vi "Filter-Get Spectrum.vi"(0 "Filter":T1 {"IIR Filter Cluster"."Forward Coefficients" format="%.4f"; "IIR Filter Cluster"."Reverse Coefficients" format="%.4f"}, 5 "Sampling Rate (Hz)":dbl, 7 "Npts":i32, 11 "error in (no error)":errorcluster) -> (4 "Filter out":T1 {"IIR Filter Cluster"."Forward Coefficients" format="%.4f"; "IIR Filter Cluster"."Reverse Coefficients" format="%.4f"}, 8 "spectrum":cdb[](array[numeric]), 15 "error out":errorcluster)   [LabVIEW 2020]
uses:
  Controls/Filter XCtl/Filter Data.ctl
  <vilib>/Analysis/2dsp.llb/Real FFT.vi
  <vilib>/Analysis/1siggen.llb/Ramp Pattern by Samples.vi
  <vilib>/Analysis/baseanly.llb/IIR Cascade Filter (DBL).vi
  Utility VIs/Math VIs/Linear to dB (array).vi
  <vilib>/Analysis/NI_AALBase.lvlib
  <vilib>/Analysis/NI_AALPro.lvlib
  Controls/Filter XCtl/Filter XCtl.xctl
panel:
  out "Magnitude":dbl[](graph)
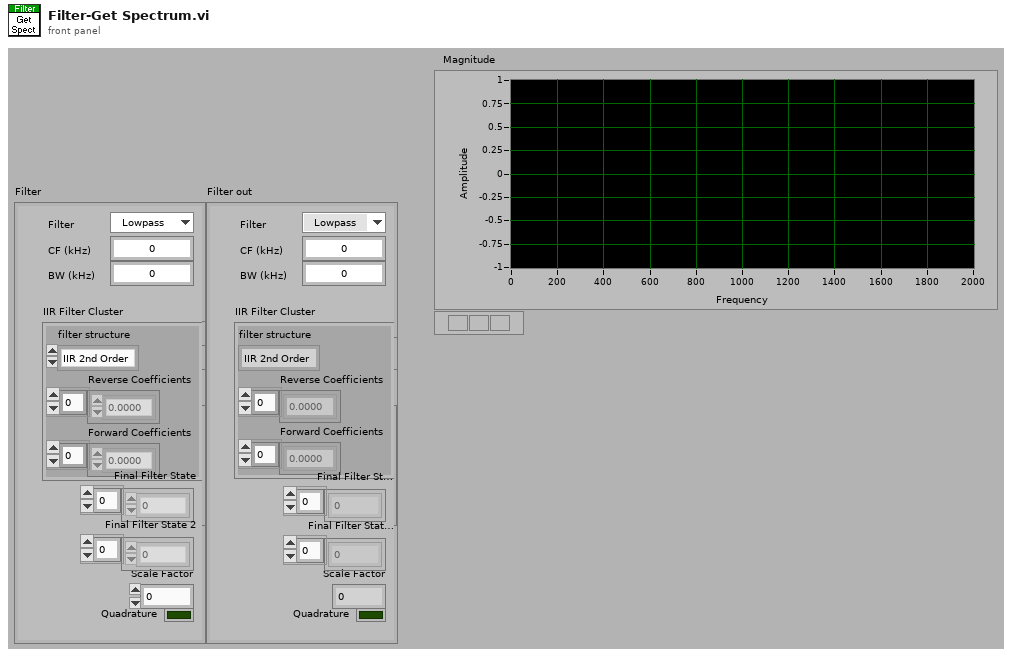
[diagram p1: front panel]
types:
  T1 = typedef "Filter XCtl.xctl/Filter Data.ctl" = cluster{"CF (kHz)":dbl, "BW (kHz)":dbl, "IIR Filter Cluster":cluster{"filter structure":enum32{"IIR 2nd Order", "IIR 4th Order"}, "Reverse Coefficients":dbl[], "Forward Coefficients":dbl[]}, "Final Filter State":dbl[], "Scale Factor":dbl, "Final Filter State 2":dbl[], "Quadrature":bool, "Type":enum16{"Lowpass", "Highpass", "Bandpass", "Bandstop", "OFF"}}
  T2 = enum16{"Lowpass", "Highpass", "Bandpass", "Bandstop", "OFF"}
  T3 = cluster{"filter structure":enum32{"IIR 2nd Order", "IIR 4th Order"}, "Reverse Coefficients":dbl[], "Forward Coefficients":dbl[]}
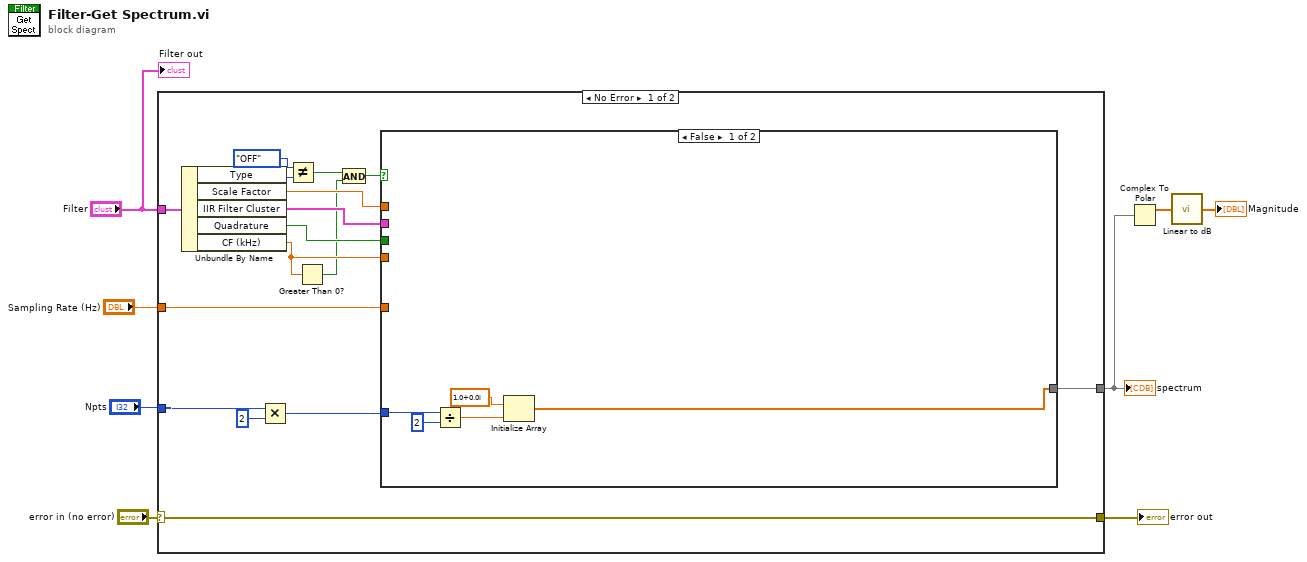
[diagram p0: block diagram]
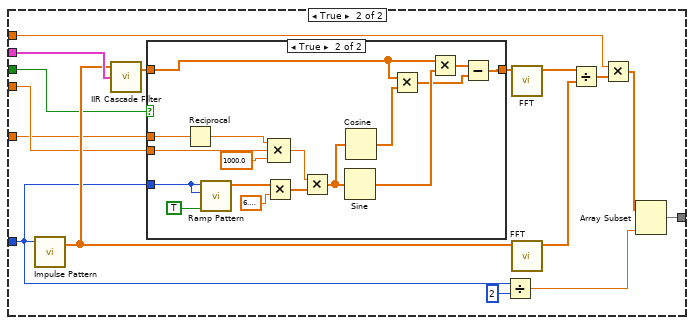
[diagram p2: hidden frame]
diagram:
  n1 = case shown="No Error" "error in (no error)" {
    selector: "error in (no error)" -> [w21 w64]
    tunnel: "Filter" -> [w23 _]
    tunnel: "Npts" -> [w16 _]
    tunnel: [w22 _] -> w5
    tunnel: [w21 w64] -> w6
    tunnel: "Sampling Rate (Hz)" -> [w15 _]
    frame No Error {
      n2 = Unbundle By Name(w23) -> ("Type"=w14:T2, "Scale Factor"=w20:dbl, "IIR Filter Cluster"=w24:T3, "Quadrature"=w17:bool, "CF (kHz)"=w10:dbl)
      n3 = Multiply(x=w16, y=2) -> (x*y=w19:i32)
      n4 = Not Equal?(x=T2."OFF", y=w14) -> (x != y?=w12:bool)
      n5 = Greater Than 0?(x=w10) -> (x > 0?=w9:bool)
      n6 = And(x=w12, y=w9) -> (x .and. y?=w11:bool)
      n7 = case shown="False" w11 {
        tunnel: w24 -> [_ w45]
        tunnel: w19 -> [w28 w30]
        tunnel: [w25 w38] -> w22
        tunnel: w20 -> [_ w36]
        tunnel: w17 -> [_ w33]
        tunnel: w10 -> [_ w32]
        tunnel: w15 -> [_ w31]
        frame False {
          n8 = Divide(x=w28, y=2) -> (x/y=w27:dbl)
          n9 = Initialize Array(cdb 1.0+0.0i ("element"), w27) -> (w25:cdb[])
        }
        frame True {
          n10 = call <vilib>:"Impulse Pattern.vi"("samples"=w30) -> ("Impulse Pattern"=w44:dbl[])  [unwired: 2 in, 1 out]
          n11 = call-poly <vilib>:"IIR Cascade Filter.vi"("IIR Filter Cluster"=w45, "X"=w44) -> ("Filtered X"=w35:dbl[])  [unwired: 1 in, 1 out]
          n12 = case shown="True" w33 {
            tunnel: w35 -> [w46 w52]
            tunnel: [w46 w51] -> w34
            tunnel: w32 -> [_ w50]
            tunnel: w30 -> [_ w49]
            tunnel: w31 -> [_ w48]
            frame False {
            }
            frame True {
              n13 = Reciprocal(x=w48) -> (1/x=w47:dbl)
              n14 = call-poly <vilib>:"Ramp Pattern.vi"("exclude end?"=TRUE, "end"=w49, "samples"=w49) -> ("Ramp Pattern"=w62:dbl[])  [unwired: 7 in, 1 out]
              n15 = Multiply(x=w62, y=6.283185307179586) -> (x*y=w61:dbl[])
              n16 = Compound Arithmetic op=MULTIPLY(w47, w50, 1000.0 ("y")) -> (w54:dbl)
              n17 = Multiply(x=w54, y=w61) -> (x*y=w59:dbl[])
              n18 = Sine(x=w59) -> (sin(x)=w60:dbl[])
              n19 = Cosine(x=w59) -> (cos(x)=w58:dbl[])
              n20 = Multiply(x=w52, y=w58) -> (x*y=w56:dbl[])
              n21 = Multiply(x=w52, y=w60) -> (x*y=w57:dbl[])
              n22 = Subtract(x=w57, y=w56) -> (x-y=w51:dbl[])
            }
          }
          n23 = Divide(x=w30, y=2) -> (x/y=w39:dbl)
          n24 = call-poly <vilib>:"FFT.vi"("X"=w34) -> ("FFT {X}"=w43:cdb[])  [unwired: 9 in, 1 out]
          n25 = call-poly <vilib>:"FFT.vi"("X"=w44) -> ("FFT {X}"=w42:cdb[])  [unwired: 9 in, 1 out]
          n26 = Divide(x=w43, y=w42) -> (x/y=w41:cdb[])
          n27 = Multiply(x=w36, y=w41) -> (x*y=w37:cdb[])
          n28 = Array Subset(array=w37, length=w39) -> (w38:cdb[])  [unwired: 1 in]
        }
      }
    }
    frame Error {
    }
  }
  "error out" <- w6
  "spectrum" <- w5
  n29 = Complex To Polar(r * e^(i*theta)=w5) -> (r=w4:dbl[])  [unwired: 1 out]
  n30 = call-poly "Linear to dB.vi"("linear"=w4) -> ("dB"=→"Magnitude":dbl[])
  "Filter out" <- "Filter"
